vi "pre_processamento.vi"() -> (0 "Tensão da Fase B":dbl[](graph), 1 "Corrente da Fase B":dbl[](graph), 2 "Corrente da Fase A":dbl[](graph), 3 "Tensão da Fase A":dbl[](graph), 4 "TimeStamp":dynamicdata(graph), 5 "Potencia B":dbl[](graph), 6 "Potencia C":dbl[](graph), 7 "Potencia A":dbl[](graph), 10 "Tensão da Fase C":dbl[](graph), 11 "Corrente da Fase C":dbl[](graph))   [LabVIEW 2020]
uses:
  <vilib>/numeric/Random Number (Range) DBL.vi
panel:
  out "result 3":dbl[](array[numeric])
  out "Array 6":dbl[](array[numeric])
  out "Array 5":dbl[](array[numeric])
  out "number 3":dbl
  out "result 2":dbl[](array[numeric])
  out "Array 4":dbl[](array[numeric])
  out "Array 3":dbl[](array[numeric])
  out "number 2":dbl
  out "result":dbl[](array[numeric])
  out "Array 2":dbl[](array[numeric])
  out "Array":dbl[](array[numeric])
  out "number":dbl
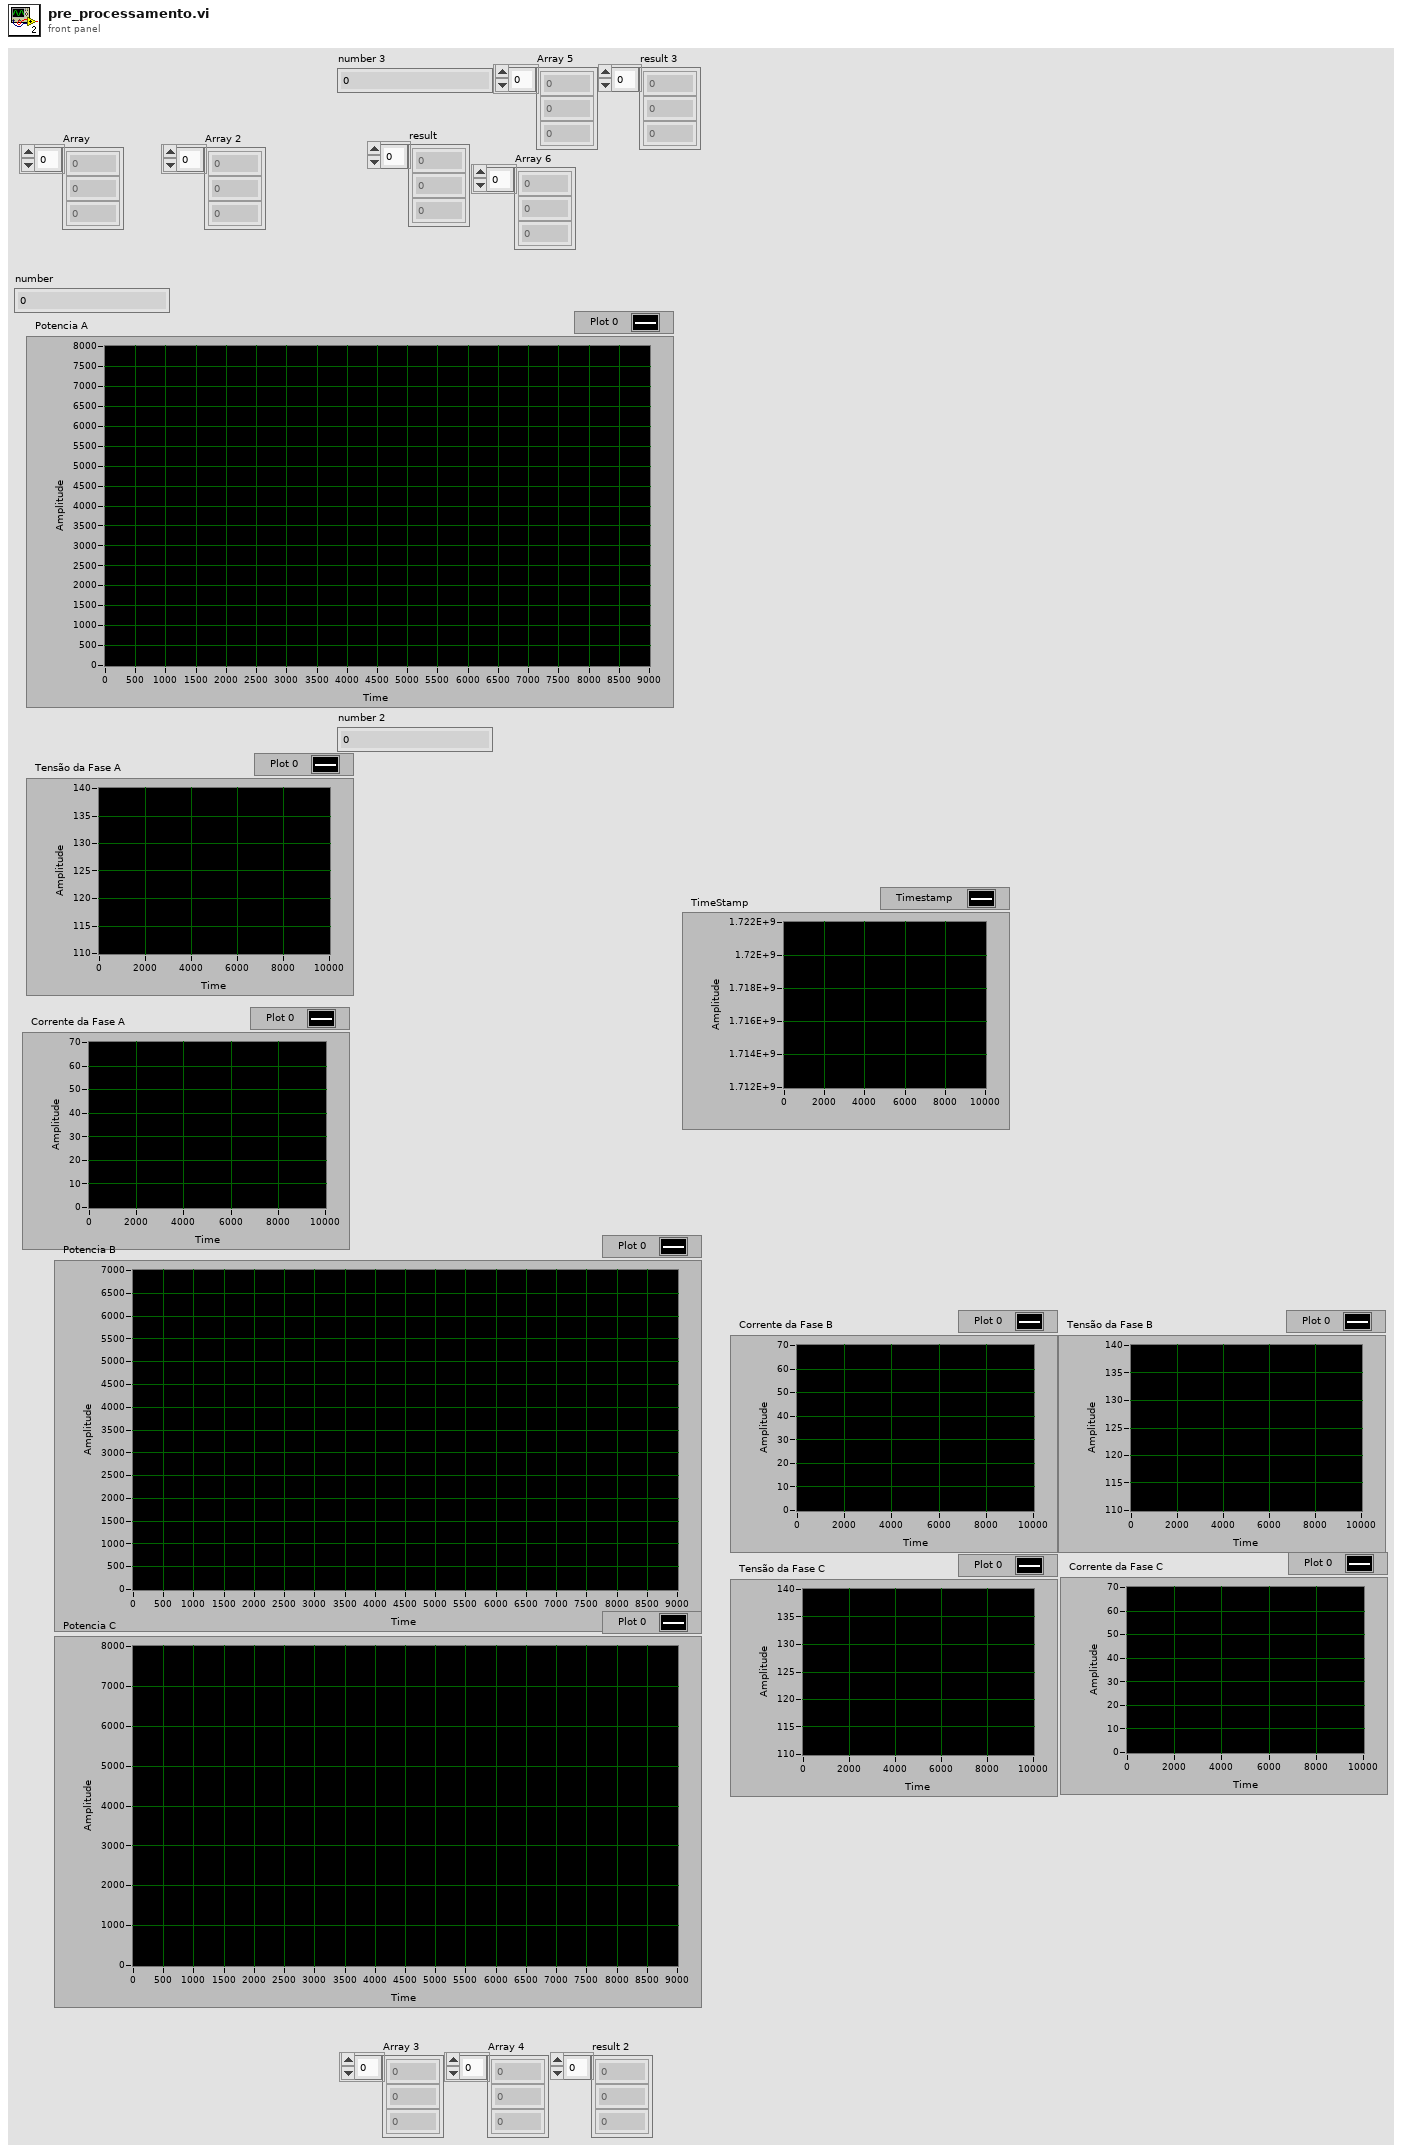
[diagram p1: front panel]
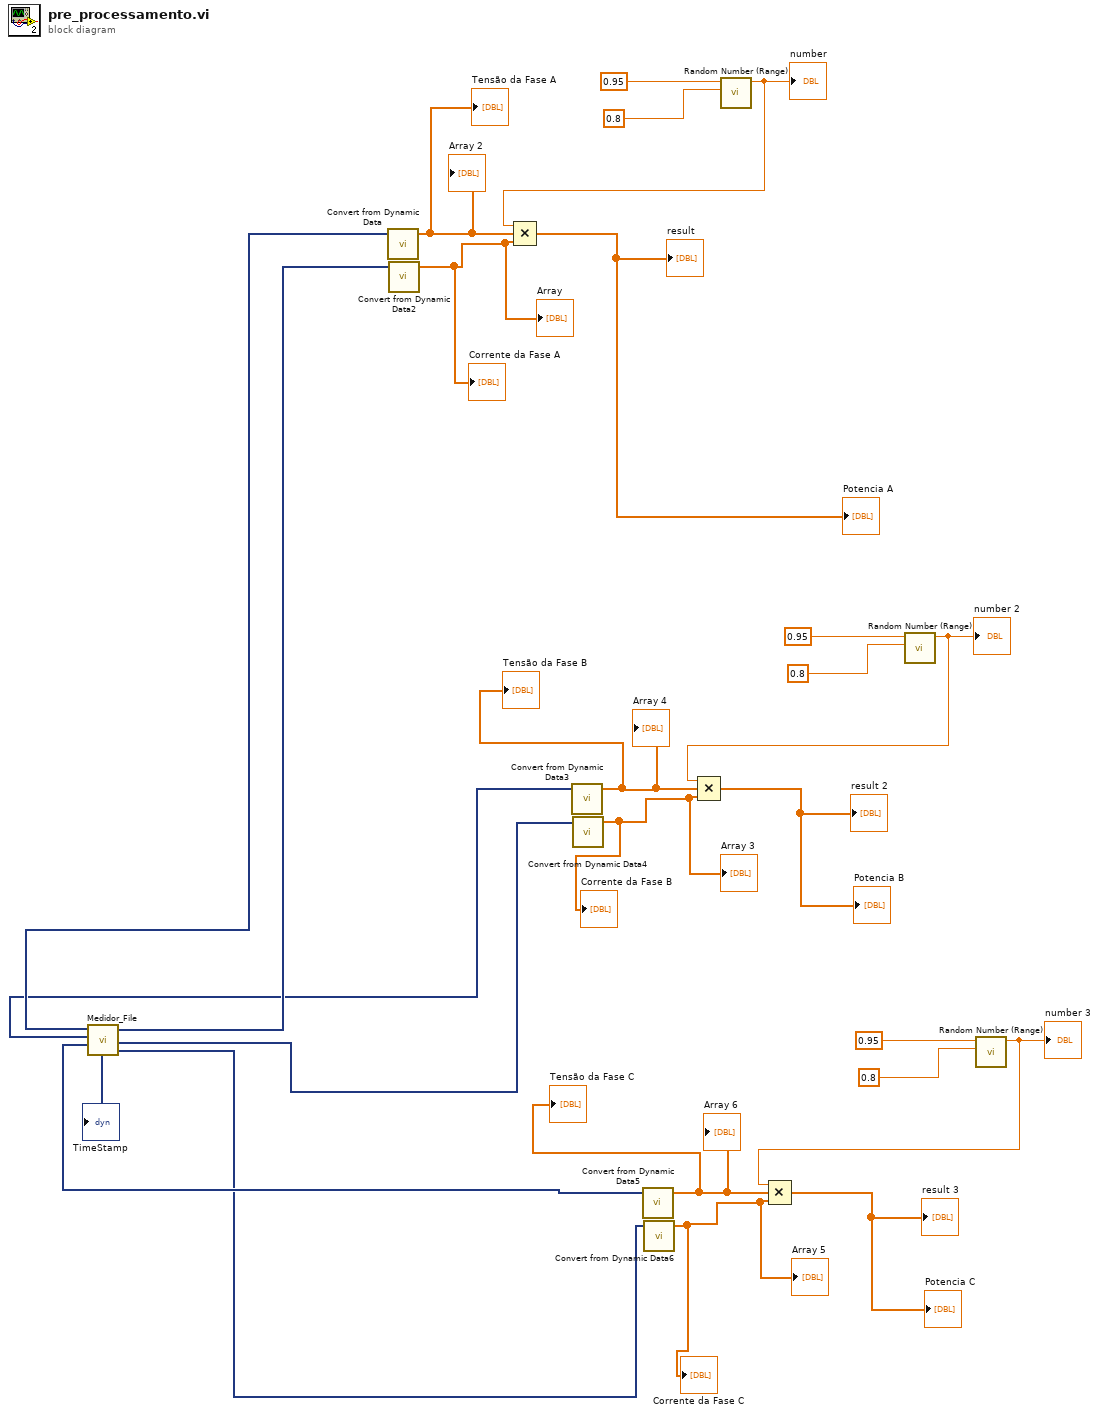
[diagram p0: block diagram]
diagram:
  n1 = call "Medidor_File.vi"() -> ("Corrente Fase C"=w10:dynamicdata, "Corrente Fase B"=w16:dynamicdata, "Corrente Fase A"=w5:dynamicdata, "TimeStamp"=→"TimeStamp":dynamicdata, "Tensão Fase C"=w11:dynamicdata, "Tensão Fase B"=w4:dynamicdata, "Tensão Fase A"=w6:dynamicdata)
  n2 = call "Convert from Dynamic Data"("Dynamic Data Type"=w6) -> ("Array"=w22:dbl[])  [unwired: 3 in]
  "Tensão da Fase A" <- w22
  "Array 2" <- w22
  n3 = call "Convert from Dynamic Data2"("Dynamic Data Type"=w5) -> ("Array"=w9:dbl[])  [unwired: 3 in]
  "Corrente da Fase A" <- w9
  "Array" <- w9
  n4 = call "Convert from Dynamic Data3"("Dynamic Data Type"=w4) -> ("Array"=w3:dbl[])  [unwired: 3 in]
  "Array 4" <- w3
  "Tensão da Fase B" <- w3
  n5 = call "Convert from Dynamic Data4"("Dynamic Data Type"=w16) -> ("Array"=w7:dbl[])  [unwired: 3 in]
  "Array 3" <- w7
  "Corrente da Fase B" <- w7
  n6 = call "Convert from Dynamic Data5"("Dynamic Data Type"=w11) -> ("Array"=w2:dbl[])  [unwired: 3 in]
  "Array 6" <- w2
  "Tensão da Fase C" <- w2
  n7 = call "Convert from Dynamic Data6"("Dynamic Data Type"=w10) -> ("Array"=w1:dbl[])  [unwired: 3 in]
  "Array 5" <- w1
  "Corrente da Fase C" <- w1
  n8 = call-poly <vilib>:"Random Number (Range).vi"("lower bound (0)"=0.8, "upper bound (100)"=0.95) -> ("number"=w23:dbl)  [unwired: 9 in]
  "number" <- w23
  n9 = Compound Arithmetic op=MULTIPLY(w23, w22, w9) -> (→"Potencia A" →"result":dbl[])
  n10 = call-poly <vilib>:"Random Number (Range).vi"("lower bound (0)"=0.8, "upper bound (100)"=0.95) -> ("number"=w18:dbl)  [unwired: 9 in]
  "number 2" <- w18
  n11 = Compound Arithmetic op=MULTIPLY(w18, w3, w7) -> (→"Potencia B" →"result 2":dbl[])
  n12 = call-poly <vilib>:"Random Number (Range).vi"("lower bound (0)"=0.8, "upper bound (100)"=0.95) -> ("number"=w13:dbl)  [unwired: 9 in]
  "number 3" <- w13
  n13 = Compound Arithmetic op=MULTIPLY(w13, w2, w1) -> (→"Potencia C" →"result 3":dbl[])
